vi "Data.Engine.Initialize.vi"(8 "error in":errorcluster, 11 "Data Access Settings":T3 {"Read"."Refs"."Data Reference" format="%.0x"; "Write"."Refs" format="%.0x"; "ReadWrite"."Refs" format="%.0x"}) -> (0 "error out":errorcluster, 3 "Data Access Engine":refnum<class "Plugin Data Access.lvclass">)   [LabVIEW 2024, in "VS Plugin Inline Async API.lvlib" / "Plugin Data Access.lvclass"]
uses:
  Plugin Data Access.lvclass
  Plugin Data Access.lvclass/Plugin Data Access.ctl
  Read/Read.lvclass
  Write/Write.lvclass
  ReadWrite/ReadWrite.lvclass
  <vilib>/NI VeriStand/Custom Device API/Data Reference.ctl
  <vilib>/NI VeriStand/Custom Device API/Custom Device API.lvlib
  <vilib>/NI VeriStand/Custom Device API/Block Data Reference.ctl
  VS Engine Abstraction/VS Engine Interface/VS Engine Interface.lvclass
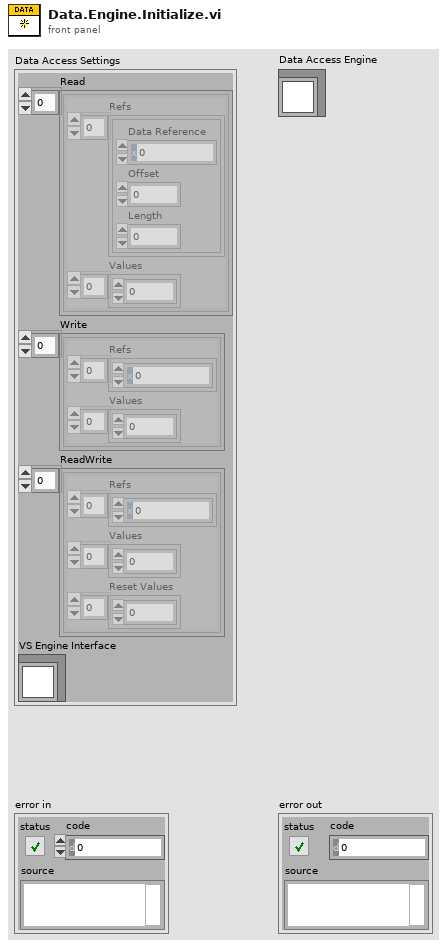
[diagram p1: front panel]
types:
  T1 = typedef "Custom Device API.lvlib/Block Data Reference.ctl" = cluster{"Data Reference":T2, "Offset":u64, "Length":u64}
  T2 = typedef "Custom Device API.lvlib/Data Reference.ctl" = i32
  T3 = cluster{"Read":cluster{"Refs":T1[], "Values":dbl[]}[], "Write":cluster{"Refs":T2[], "Values":dbl[]}[], "ReadWrite":cluster{"Refs":T2[], "Values":dbl[], "Reset Values":dbl[]}[], "VS Engine Interface":refnum<class "VS Engine Interface.lvclass">}
  T4 = cluster{"Refs":T2[], "Values":dbl[], "Reset Values":dbl[]}[]
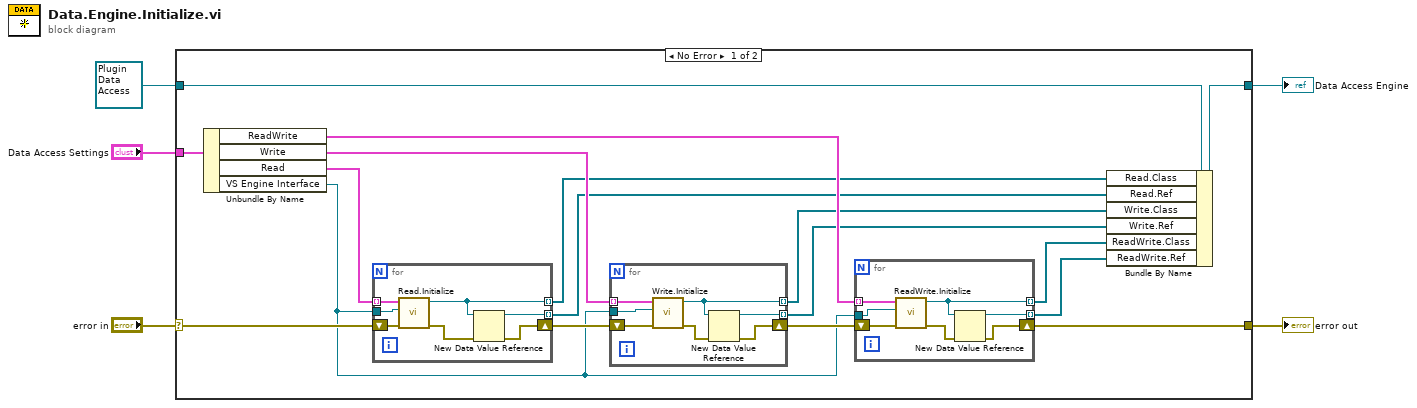
[diagram p0: block diagram]
diagram:
  n1 = case shown="No Error" "error in" {
    selector: "error in" -> [w22 w45]
    tunnel: [w19 w45] -> w4
    tunnel: [w12 w44] -> w2
    tunnel: refnum<class "Plugin Data Access.lvclass"> refnum ("Data Access API.lvlib:Data Access API.lvclass") -> [w7 w44]
    tunnel: "Data Access Settings" -> [w8 _]
    frame No Error {
      n2 = Unbundle By Name(w8) -> ("ReadWrite"=w16:T4, "Write"=w17:cluster{"Refs":T2[], "Values":dbl[]}[], "Read"=w18:cluster{"Refs":T1[], "Values":dbl[]}[], "VS Engine Interface"=w6:refnum<class "VS Engine Interface.lvclass">)
      n3 = for {
        tunnel: w18 -> [w40] mode=indexing
        shift-right: [w41] -> w21
        shift-left: w22 -> [w43]
        tunnel: [w38] -> w13 mode=indexing
        tunnel: [w39] -> w9 mode=indexing
        tunnel: w6 -> [w37]
        n4 = call "Read.Initialize.vi"("error in"=w43, "VS Engine Interface"=w37, "Settings"=w40) -> ("error out"=w42:errorcluster, "Read out"=w38:refnum<class "Read.lvclass">)  [unwired: 7 in]
        n5 = New Data Value Reference(data value=w38, error in=w42) -> (data value reference=w39:refnum<data-value>, error out=w41:errorcluster)
      }
      n6 = for {
        tunnel: w17 -> [w33] mode=indexing
        shift-right: [w34] -> w20
        shift-left: w21 -> [w36]
        tunnel: [w32] -> w14 mode=indexing
        tunnel: [w31] -> w10 mode=indexing
        tunnel: w6 -> [w30]
        n7 = call "Write.Initialize.vi"("error in"=w36, "VS Engine Interface"=w30, "Settings"=w33) -> ("error out"=w35:errorcluster, "Write out"=w32:refnum<class "Write.lvclass">)  [unwired: 7 in]
        n8 = New Data Value Reference(data value=w32, error in=w35) -> (data value reference=w31:refnum<data-value>, error out=w34:errorcluster)
      }
      n9 = for {
        tunnel: w16 -> [w26] mode=indexing
        shift-right: [w27] -> w19
        shift-left: w20 -> [w29]
        tunnel: [w25] -> w15 mode=indexing
        tunnel: [w24] -> w11 mode=indexing
        tunnel: w6 -> [w23]
        n10 = call "ReadWrite.Initialize.vi"("error in"=w29, "VS Engine Interface"=w23, "Settings"=w26) -> ("error out"=w28:errorcluster, "ReadWrite out"=w25:refnum<class "ReadWrite.lvclass">)  [unwired: 7 in]
        n11 = New Data Value Reference(data value=w25, error in=w28) -> (data value reference=w24:refnum<data-value>, error out=w27:errorcluster)
      }
      n12 = Bundle By Name(cluster=w7, "Read.Class"=w13, "Read.Ref"=w9, "Write.Class"=w14, "Write.Ref"=w10, "ReadWrite.Class"=w15, "ReadWrite.Ref"=w11) -> (w12:refnum<class "Plugin Data Access.lvclass">)
    }
    frame Error {
    }
  }
  "error out" <- w4
  "Data Access Engine" <- w2
